vi "UMLEditor SendMessageToWizard.vi"(1 "MessageType":string, 2 "MessageData":string, 3 "AllowErrorPopup(True)":bool=TRUE, 5 "error in (no error)":errorcluster) -> (15 "Error":bool, 19 "error out":errorcluster)   [LabVIEW 2012]
doc: "Gets current diagram values"
uses:
  <resource>/Framework/Providers/Open_GDS/UML/UMLEditor/UMLEditor_StoredPathes.ctl
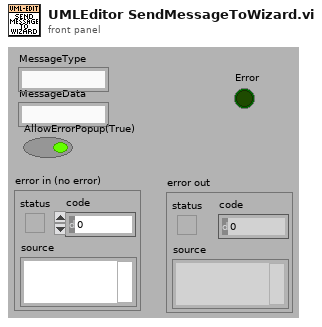
[diagram p1: front panel]
types:
  T1 = typedef "UMLEditor_StoredPathes.ctl" = enum16{"LastSearchPath", "QueuedArrayStateVI", "ClassBasePath", "ViTemplatePath", "ApplicationTemplatePath", "IniFilePath", "WizDir", "RevPlugInPath"}
  T2 = enum32{"Bad", "Idle", "Run top level", "Running"}
  T3 = cluster{"Sender":string, "MessageType":string, "Timestamp":dbl, "Message":string, "Messages":string[]}
  T4 = typedef "Queue RefNum" = refnum<k1>
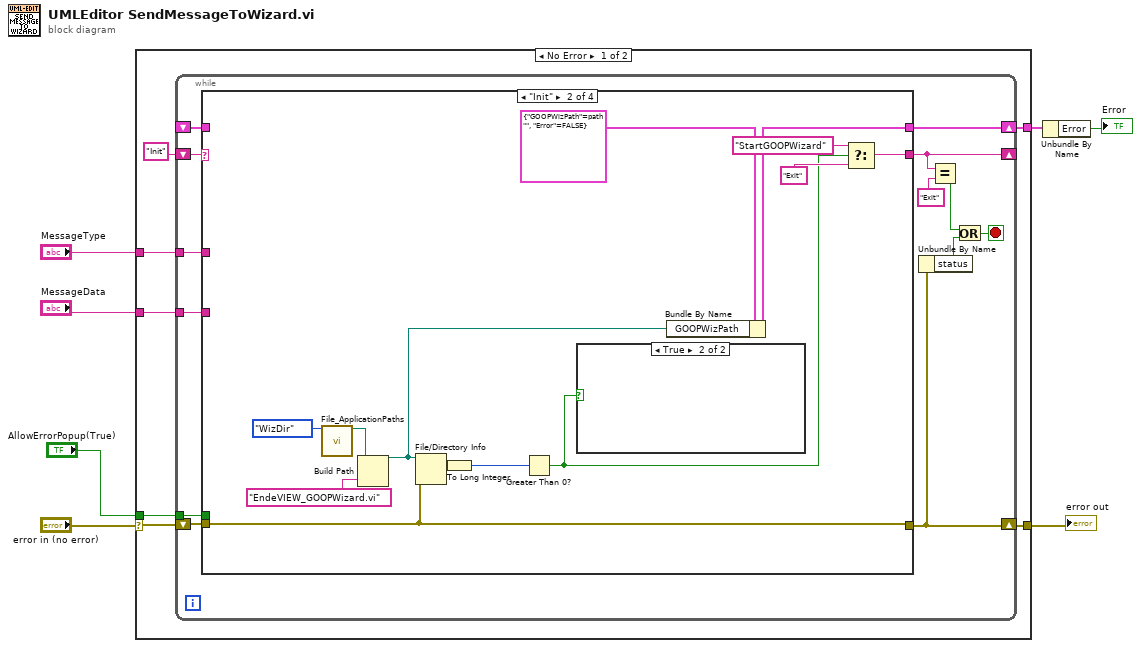
[diagram p0: block diagram]
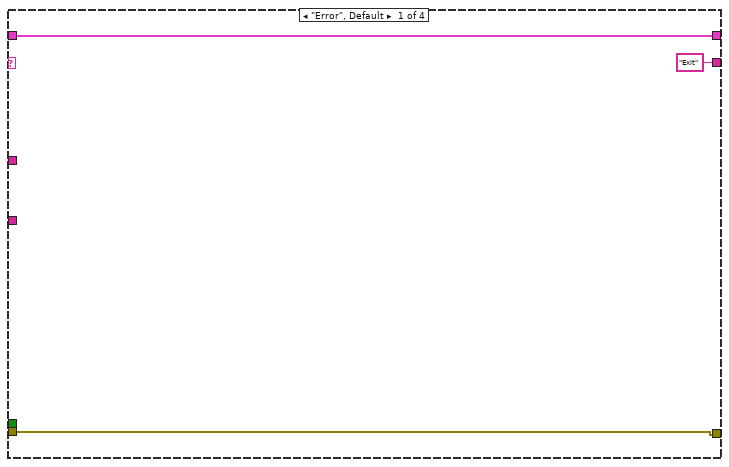
[diagram p2: hidden frame]
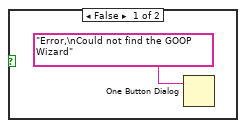
[diagram p3: hidden frame]
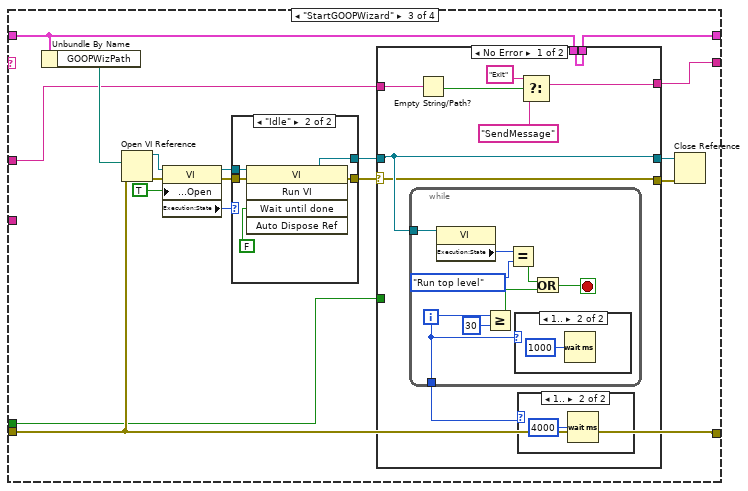
[diagram p4: hidden frame]
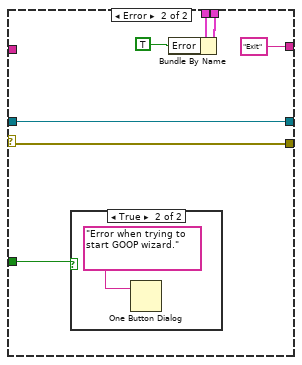
[diagram p7: hidden frame]
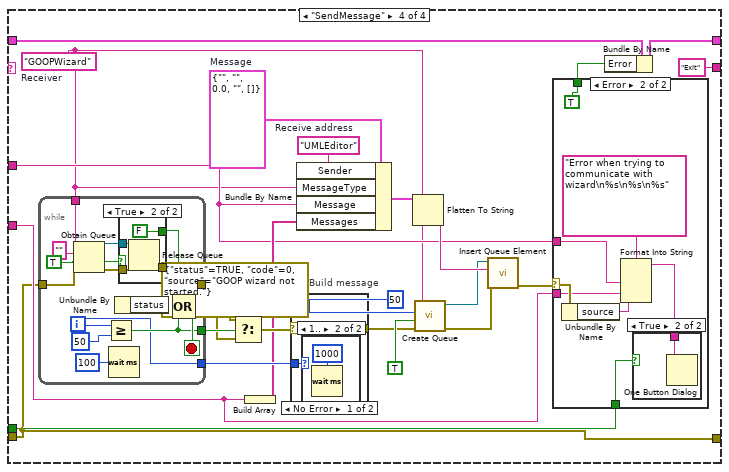
[diagram p10: hidden frame]
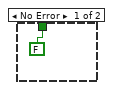
[diagram p14: hidden frame]
diagram:
  n1 = case shown="No Error" "error in (no error)" {
    selector: "error in (no error)" -> [w12 w156]
    tunnel: [w13 w156] -> w6
    tunnel: "MessageData" -> [w11 _]
    tunnel: "MessageType" -> [w10 _]
    tunnel: [w9 _] -> w3
    tunnel: "AllowErrorPopup(True)" -> [w8 _]
    frame No Error {
      n2 = while {
        shift-right: [w23] -> w13
        shift-left: w12 -> [w27]
        shift-right: [w21] -> _
        shift-left: "Init" -> [w26]
        shift-right: [w25] -> w9
        shift-left: _ -> [w24]
        tunnel: w11 -> [w17]
        tunnel: w10 -> [w16]
        tunnel: w8 -> [w15]
        stop <- w18 stop-if-true
        n3 = case shown="\"Init\"" w26 {
          tunnel: w27 -> [w28 w37 w54 w107]
          tunnel: [w28 w37 w54 w107] -> w23
          tunnel: [w29 w35 w45 w114] -> w25
          tunnel: ["Exit" w43 w53 "Exit" ("y")] -> w21
          tunnel: w24 -> [w29 _ w46 w115]
          tunnel: w17 -> [_ _ _ w116]
          tunnel: w16 -> [_ _ w48 w98]
          tunnel: w15 -> [_ _ w47 w112]
          frame "Error", Default {
          }
          frame "Init" {
            n4 = call <resource>:"File_ApplicationPaths.vi"("PathName"=UMLEditor_StoredPathes."WizDir" ("UMLPathes")) -> ("Path Out"=w32:path)  [unwired: 3 in, 15 out]
            n5 = Build Path(base path=w32, name or relative path="EndeVIEW_GOOPWizard.vi") -> (appended path=w40:path)
            n6 = File/Directory Info(path=w40, error in=w37) -> (size=w31:i64)  [unwired: 6 out]
            n7 = To Long Integer(number=w31) -> (32bit integer=w41:i32)
            n8 = Greater Than 0?(x=w41) -> (x > 0?=w38:bool)
            n9 = case shown="True" w38 {
              frame False {
                n10 = One Button Dialog(message="Error,\nCould not find the GOOP Wizard") -> ()  [unwired: 2 out]
              }
              frame True {
              }
            }
            n11 = Bundle By Name(cluster=cluster{"GOOPWizPath":path, "Error":bool} {"GOOPWizPath"=path "", "Error"=FALSE}, "GOOPWizPath"=w40) -> (w35:cluster{"GOOPWizPath":path, "Error":bool})
            n12 = Select(t="StartGOOPWizard", s=w38, f="Exit" ("y")) -> (s? t:f=w43:string)
          }
          frame "StartGOOPWizard" {
            n13 = Unbundle By Name(w46) -> ("GOOPWizPath"=w55:path)
            n14 = Open VI Reference(vi path=w55, error in (no error)=w54) -> (vi reference=w61:refnum<vi>, error out=w60:errorcluster)  [unwired: 4 out]
            n15 = property class="VI"(reference=w61, error in=w60, "Front Panel Window:Open"=TRUE) -> (reference out=w57:refnum<vi>, error out=w56:errorcluster, "Execution:State"=w58:T2)
            n16 = case shown="\"Idle\"" w58 {
              tunnel: w57 -> [w89 w94]
              tunnel: w56 -> [w90 w95]
              tunnel: [w90 w93] -> w52
              tunnel: [w89 w92] -> w51
              frame Default {
              }
              frame "Idle" {
                n17 = invoke class="VI" method="Run VI"(reference=w94, error in=w95, "Wait until done"=FALSE) -> (reference out=w92:refnum<vi>, error out=w93:errorcluster)  [unwired: 2 in, 3 out]
              }
            }
            n18 = case shown="No Error" w52 {
              selector: w52 -> [w69 w85]
              tunnel: [w64 "Exit" ("y")] -> w53
              tunnel: w51 -> [w70 w86]
              tunnel: [w70 w86] -> w50
              tunnel: [w69 w85] -> w49
              tunnel: w48 -> [w68 _]
              tunnel: w47 -> [_ w84]
              tunnel: w46 -> [w62 w83]
              tunnel: [w62 w82] -> w45
              frame No Error {
                n19 = while {
                  tunnel: w70 -> [w79]
                  tunnel: [w72] -> w63
                  i -> [w72]
                  stop <- w73 stop-if-true
                  n20 = property class="VI"(reference=w79) -> ("Execution:State"=w78:T2)  [unwired: 1 in, 2 out]
                  n21 = Greater Or Equal?(x=w72, y=30) -> (x >= y?=w74:bool)
                  n22 = Equal?(x=w78, y=T2."Run top level" ("Execution:State")) -> (x = y?=w75:bool)
                  n23 = case shown="1.." w72 {
                    frame 0, Default {
                    }
                    frame 1.. {
                      n24 = Wait (ms)(milliseconds to wait=u32 1000) -> ()  [unwired: 1 out]
                    }
                  }
                  n25 = Or(x=w75, y=w74) -> (x .or. y?=w73:bool)
                }
                n26 = Empty String/Path?(string/path=w68) -> (empty?=w67:bool)
                n27 = case shown="1.." w63 {
                  frame 0, Default {
                  }
                  frame 1.. {
                    n28 = Wait (ms)(milliseconds to wait=u32 4000) -> ()  [unwired: 1 out]
                  }
                }
                n29 = Select(t="Exit" ("y"), s=w67, f="SendMessage" ("y")) -> (s? t:f=w64:string)
              }
              frame Error {
                n30 = case shown="True" w84 {
                  frame False {
                  }
                  frame True {
                    n31 = One Button Dialog(message="Error when trying to start GOOP wizard.") -> ()  [unwired: 2 out]
                  }
                }
                n32 = Bundle By Name(cluster=w83, "Error"=TRUE) -> (w82:cluster{"GOOPWizPath":path, "Error":bool})
              }
            }
            n33 = Close Reference(reference=w50, error in (no error)=w49) -> ()  [unwired: 1 out]
          }
          frame "SendMessage" {
            w106 = T3 {"Sender"="", "MessageType"="", "Timestamp"=0.0, "Message"="", "Messages"=[]}  # Message
            w97 = "GOOPWizard"  # Receiver
            w96 = "UMLEditor"  # Receive address
            # "Build message"
            n34 = while {
              tunnel: w107 -> [w128]
              tunnel: [w127] -> w118
              tunnel: w97 -> [w125]
              tunnel: [w135] -> w119
              tunnel: [w134] -> w110
              i -> [w134]
              stop <- w137 stop-if-true
              n35 = Obtain Queue(name (unnamed)=w125, element data type="", create if not found? (T)=TRUE ("return existing (F)"), error in (no error)=w128) -> (queue out=w130:refnum<queue>, created new?=w133:bool, error out=w131:errorcluster)  [unwired: 1 in]
              n36 = Greater Or Equal?(x=w134, y=50) -> (x >= y?=w135:bool)
              n37 = Wait (ms)(milliseconds to wait=u32 100) -> ()  [unwired: 1 out]
              n38 = case shown="True" w133 {
                tunnel: w131 -> [w141 w145]
                tunnel: w130 -> [_ w144]
                tunnel: [w141 w143] -> w127
                tunnel: [TRUE FALSE] -> w126
                frame False {
                }
                frame True {
                  n39 = Release Queue(queue=w144, error in (no error)=w145) -> (error out=w143:errorcluster)  [unwired: 3 out]
                }
              }
              n40 = Unbundle By Name(w127) -> ("status"=w136:bool)
              n41 = Compound Arithmetic op=OR(w126, w136, w135) -> (w137:bool)
            }
            n42 = Select(t=errorcluster {"status"=TRUE, "code"=0, "source"="GOOP wizard not started."}, s=w119, f=w118) -> (s? t:f=w111:errorcluster)
            n43 = Build Array(w116) -> (w99:string[])
            n44 = case shown="No Error" w111 {
              selector: w111 -> [w122 w124]
              tunnel: [w122 w124] -> w100
              tunnel: w110 -> [w121 _]
              frame No Error {
                n45 = case shown="1.." w121 {
                  frame 0, Default {
                  }
                  frame 1.. {
                    n46 = Wait (ms)(milliseconds to wait=u32 1000) -> ()  [unwired: 1 out]
                  }
                }
              }
              frame Error {
              }
            }
            n47 = Bundle By Name(cluster=w106, "Sender"=w96, "MessageType"=w97, "Message"=w98, "Messages"=w99) -> (w104:T3)
            n48 = Flatten To String(anything=w104) -> (data string=w103:string)  [unwired: 1 in, 4 out]
            n49 = call <vilib>:"Create Queue.vi"("error in (no error)"=w100, "return existing (F)"=TRUE, "size (unbounded)"=50, "name (unnamed)"=w97) -> ("error out"=w101:errorcluster, "queue out"=w102:T4)  [unwired: 2 out]
            n50 = call <vilib>:"Insert Queue Element.vi"("error in (no error)"=w101, "queue element"=w103, "queue"=w102) -> ("error out"=w105:errorcluster)  [unwired: 2 in, 4 out]
            n51 = case shown="Error" w105 {
              selector: w105 -> [_ w154]
              tunnel: w98 -> [_ w150]
              tunnel: w116 -> [_ w149]
              tunnel: [FALSE TRUE] -> w113
              tunnel: w112 -> [_ w147]
              frame No Error {
              }
              frame Error {
                n52 = Unbundle By Name(w154) -> ("source"=w151:string)
                n53 = Format Into String(format string="Error when trying to communicate with  wizard\n%s\n%s\n%s" ("message"), w150, w149, w151) -> (resulting string=w152:string)  [unwired: 2 in, 1 out]
                n54 = case shown="True" w147 {
                  tunnel: w152 -> [_ w155]
                  frame False {
                  }
                  frame True {
                    n55 = One Button Dialog(message=w155) -> ()  [unwired: 2 out]
                  }
                }
              }
            }
            n56 = Bundle By Name(cluster=w115, "Error"=w113) -> (w114:cluster{"GOOPWizPath":path, "Error":bool})
          }
        }
        n57 = Unbundle By Name(w23) -> ("status"=w22:bool)
        n58 = Equal?(x=w21, y="Exit") -> (x = y?=w19:bool)
        n59 = Or(x=w19, y=w22) -> (x .or. y?=w18:bool)
      }
    }
    frame Error {
    }
  }
  "error out" <- w6
  n60 = Unbundle By Name(w3) -> ("Error"=→"Error":bool)
